vi "Get Incrementing Class Name.vi"() -> (3 "String":string)   [LabVIEW 2020, in "Process Generation.lvlib" / "New Class Dialog.lvclass"]
uses:
  New Class Dialog.lvclass
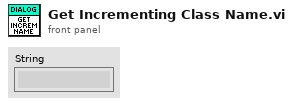
[diagram p1: front panel]
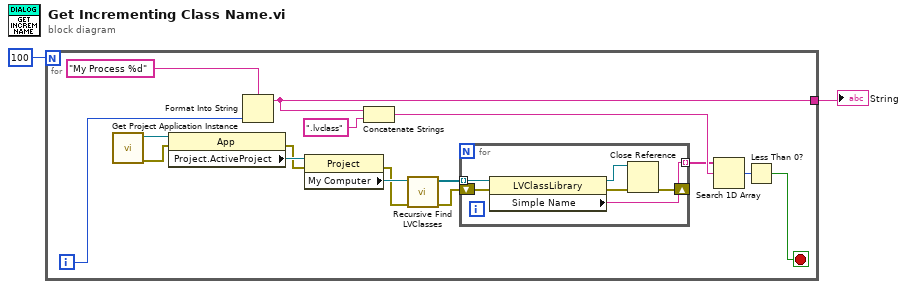
[diagram p0: block diagram]
diagram:
  n1 = for {
    N: 100 -> [_]
    tunnel: [w16] -> w2
    i -> [w17]
    stop <- w13 stop-if-true
    n2 = call "Get Project Application Instance.vi"() -> ("error out"=w7:errorcluster, "Application out"=w8:refnum<vi>)  [unwired: 10 in]
    n3 = property class="App"(reference=w8, error in=w7) -> (error out=w6:errorcluster, "Project.ActiveProject"=w12:refnum<vi>)  [unwired: 1 out]
    n4 = Format Into String(format string="My Process %d", w17) -> (resulting string=w16:string)  [unwired: 2 in, 1 out]
    n5 = property class="Project"(reference=w12, error in=w6) -> (error out=w5:errorcluster, "My Computer"=w9:refnum<vi>)  [unwired: 1 out]
    n6 = Concatenate Strings(w16, ".lvclass" ("string")) -> (w15:string)
    n7 = call "Recursive Find LVClasses.vi"("error in (no error)"=w5, "reference"=w9) -> ("error out"=w4:errorcluster, "Class References"=w10:refnum<vi>[])  [unwired: 8 in]
    n8 = for {
      tunnel: w10 -> [w24] mode=indexing
      tunnel: [w23] -> w11 mode=indexing
      shift-right: [w19] -> _
      shift-left: w4 -> [w22]
      n9 = property class="LVClassLibrary"(reference=w24, error in=w22) -> (reference out=w20:refnum<vi>, error out=w21:errorcluster, "Simple Name"=w23:string)
      n10 = Close Reference(reference=w20, error in (no error)=w21) -> (error out=w19:errorcluster)
    }
    n11 = Search 1D Array(1D array=w11, element=w15) -> (index of element=w14:i32)  [unwired: 1 in]
    n12 = Less Than 0?(x=w14) -> (x < 0?=w13:bool)
  }
  "String" <- w2
